vi "RemoveTabsFromText.vi"(11 "Tabbed Text":string) -> (3 "Non-Tabbed Text":string)   [LabVIEW 2012, in "Virtual-PGA.lvlib"]
uses:
  Virtual-PGA.lvlib
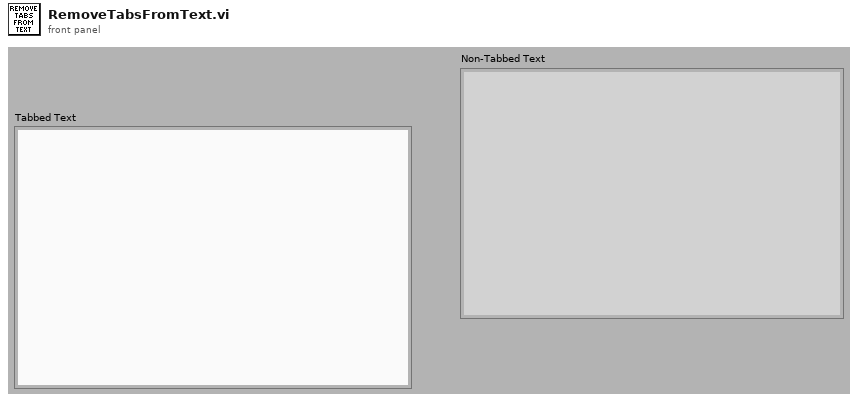
[diagram p1: front panel]
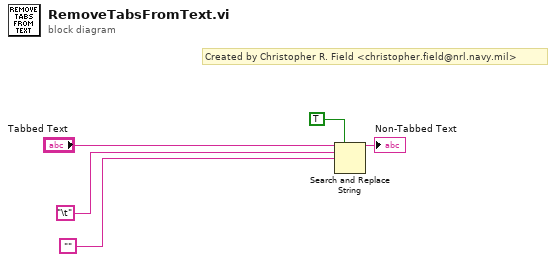
[diagram p0: block diagram]
diagram:
  # "Created by Christopher R. Field <christopher.field@nrl.navy.mil>"
  n1 = Search and Replace String(replace all?=TRUE ("replace all? (F)"), input string="Tabbed Text", search string="\t", replace string="") -> (result string=→"Non-Tabbed Text":string)  [unwired: 4 in, 3 out]
